vi "getNeighbors.vi"(10 "Nodes":cluster{"Weight":dbl, "Row":dbl, "Col":dbl}[][](array[cluster]), 11 "Node":cluster{"Weight":dbl, "Row":dbl, "Col":dbl}) -> (3 "neighbors":cluster{"Weight":dbl, "Row":dbl, "Col":dbl}[](array[cluster]))   [LabVIEW 2014]
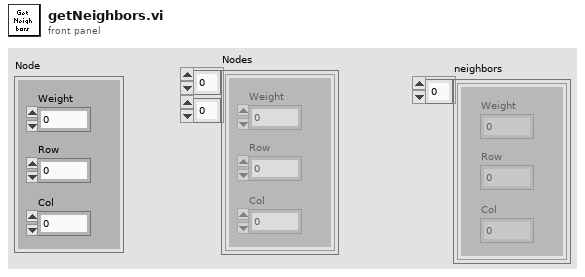
[diagram p1: front panel]
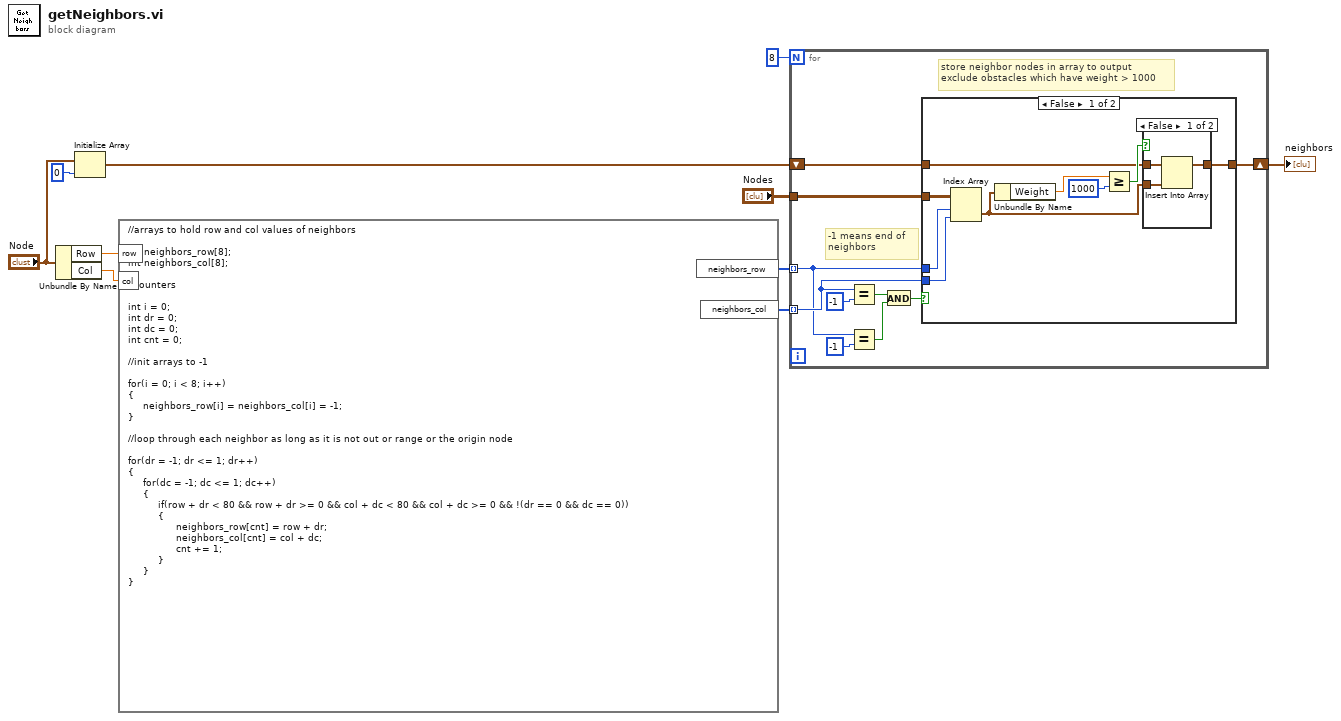
[diagram p0: block diagram]
diagram:
  n1 = Unbundle By Name("Node") -> ("Row"=w10:dbl, "Col"=w9:dbl)
  n2 = Initialize Array("Node", 0) -> (w2:cluster{"Weight":dbl, "Row":dbl, "Col":dbl}[])
  n3 = formula code="//arrays to hold row and col values of neighbors\n\nint neighbors_row[8];\nint neighbors_col[8];\n\n//counters\n\nint i = 0;\nint dr = 0;\nint dc = 0;\nint cnt = 0;\n\n//init arrays to -1\n\nfor(i = 0; i < 8; i++)\n{\n     neighbors_row[i] = neighbors_col[i] = -1;\n}\n\n//loop through each neighbor as long as it is not out or range or the origin node\n\nfor(dr = -1; dr <= 1; dr++)\n{\n     for(dc = -1; dc <= 1; dc++)\n     {\n          if(row + dr < 80 && row + dr >= 0 && col + dc < 80 && col + dc >= 0 && !(dr == 0 && dc == 0))\n          {\n                neighbors_row[cnt] = row + dr;\n                neighbors_col[cnt] = col + dc;\n                cnt += 1; \n          }\n     }\n}"("row"=w10, "col"=w9) -> ("neighbors_row"=w7:i32[], "neighbors_col"=w6:i32[])
  n4 = for {
    N: 8 -> [_]
    tunnel: w7 -> [w13] mode=indexing
    tunnel: w6 -> [w14] mode=indexing
    shift-right: [w12] -> w1
    shift-left: w2 -> [w11]
    tunnel: "Nodes" -> [w15]
    # "-1 means end of \nneighbors"
    # "store neighbor nodes in array to output\nexclude obstacles which have weight > 1000"
    n5 = Equal?(x=w14, y=-1) -> (x = y?=w18:bool)
    n6 = Equal?(x=w13, y=-1) -> (x = y?=w17:bool)
    n7 = And(x=w18, y=w17) -> (x .and. y?=w16:bool)
    n8 = case shown="False" w16 {
      tunnel: w15 -> [w29 _]
      tunnel: w14 -> [w27 _]
      tunnel: w13 -> [w28 _]
      tunnel: [w21 w34] -> w12
      tunnel: w11 -> [w22 w34]
      frame False {
        n9 = Index Array(array=w29, index (row)=w28, index (col)=w27) -> (element=w23:cluster{"Weight":dbl, "Row":dbl, "Col":dbl})
        n10 = Unbundle By Name(w23) -> ("Weight"=w26:dbl)
        n11 = Greater Or Equal?(x=w26, y=1000) -> (x >= y?=w24:bool)
        n12 = case shown="False" w24 {
          tunnel: w23 -> [w32 _]
          tunnel: w22 -> [w31 w33]
          tunnel: [w30 w33] -> w21
          frame False {
            n13 = Insert Into Array(array=w31, new element=w32) -> (w30:cluster{"Weight":dbl, "Row":dbl, "Col":dbl}[])  [unwired: 1 in]
          }
          frame True {
          }
        }
      }
      frame True {
      }
    }
  }
  "neighbors" <- w1
